vi "Encrypt.vi"(10 "String":string, 11 "Encryption in":refnum<class "Encryption.lvclass">) -> (2 "Encrypted String":string, 3 "Encryption out":refnum<class "Encryption.lvclass">)   [LabVIEW 2013, in "SMOConfig.lvlib" / "Encryption.lvclass"]
uses:
  Encryption.lvclass
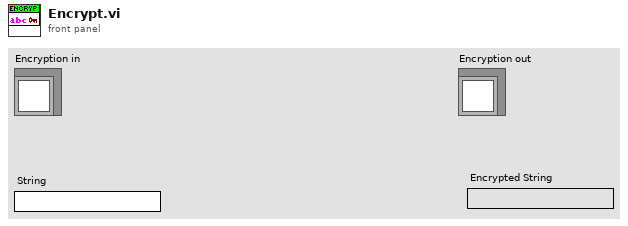
[diagram p1: front panel]
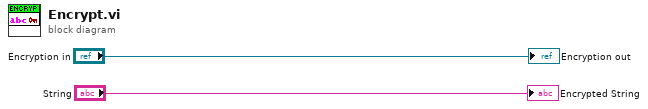
[diagram p0: block diagram]
diagram:
  "Encryption out" <- "Encryption in"
  "Encrypted String" <- "String"
